vi "New dotNET Socket Listener.vi"(8 "error in (no error)":errorcluster) -> (0 "error out":errorcluster, 3 "dotNET Listener out":refnum<class "dotNET Listener.lvclass">)   [LabVIEW 2013, in "dotNET SSL Socket.lvlib" / "dotNET Listener.lvclass"]
uses:
  dotNET Listener.lvclass
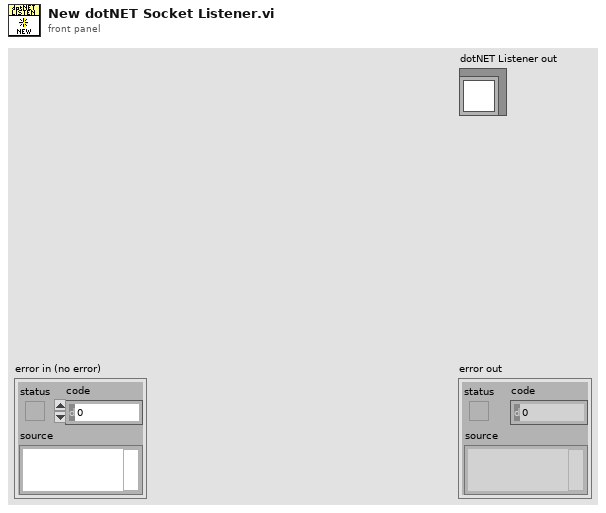
[diagram p1: front panel]
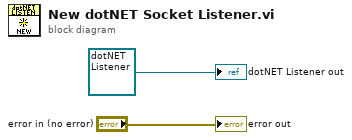
[diagram p0: block diagram]
diagram:
  "error out" <- "error in (no error)"
  "dotNET Listener out" <- refnum<class "dotNET Listener.lvclass"> refnum ("dotNET Listener in")
